vi "ReadValue_Control2.vi"(11 "reference":refnum<vi>) -> (2 "value":T1)   [LabVIEW 2012]
uses:
  Typedefs/Control 2.ctl
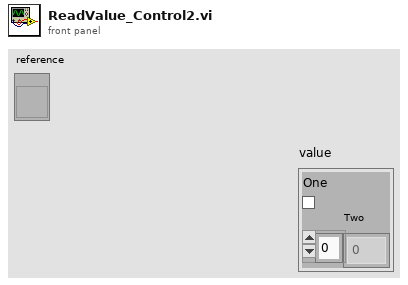
[diagram p1: front panel]
types:
  T1 = typedef "Control 2.ctl" = cluster{"One":bool, "Two":i32[]}
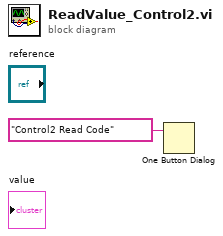
[diagram p0: block diagram]
diagram:
  n1 = One Button Dialog(message="Control2 Read Code" ("button name (\"OK\")")) -> ()  [unwired: 1 in, 1 out]
